vi "DIO tester.vi"() -> ()   [LabVIEW 2013]
uses:
  <vilib>/rvi/Emulation/niFpgaSctlEmulationGetInTimedLoop.vi
  <vilib>/rvi/Emulation/niFpgaEmulationReportErrorSimple.vi
  <vilib>/rvi/Emulation/niFpgaGetClockAttributes.vi
  <vilib>/rvi/eio/common/nirviEmuTemplateMethod_errors.vi
  <vilib>/rvi/Emulation/niFpgaCriticalErrorInLSC.vi
  <vilib>/rvi/Emulation/niFpgaProcessEmulError.vi
  <vilib>/eio/EIONode/EIONode.xnode
panel:
  in  "WE":bool
  in  "IO Module\\DIO Port 0 WE":bool
  out "Row bits":u8 format="%.0b"
  out "Column bits":u8 format="%.0b"
  out "bit9":bool
  out "bit8":bool
  out "Port1":u8 format="%.0b"
  out "Port0":u8 format="%.0b"
  in  "auto":bool
  out "Column":u16
  out "Row":u16
  in  "10thIndex":u8
  in  "ActiveLedIndex":u16
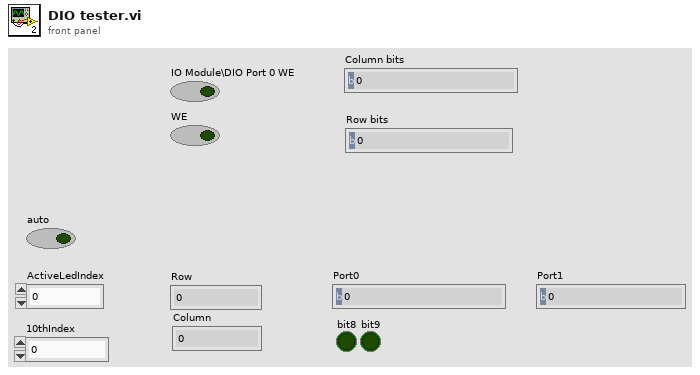
[diagram p1: front panel]
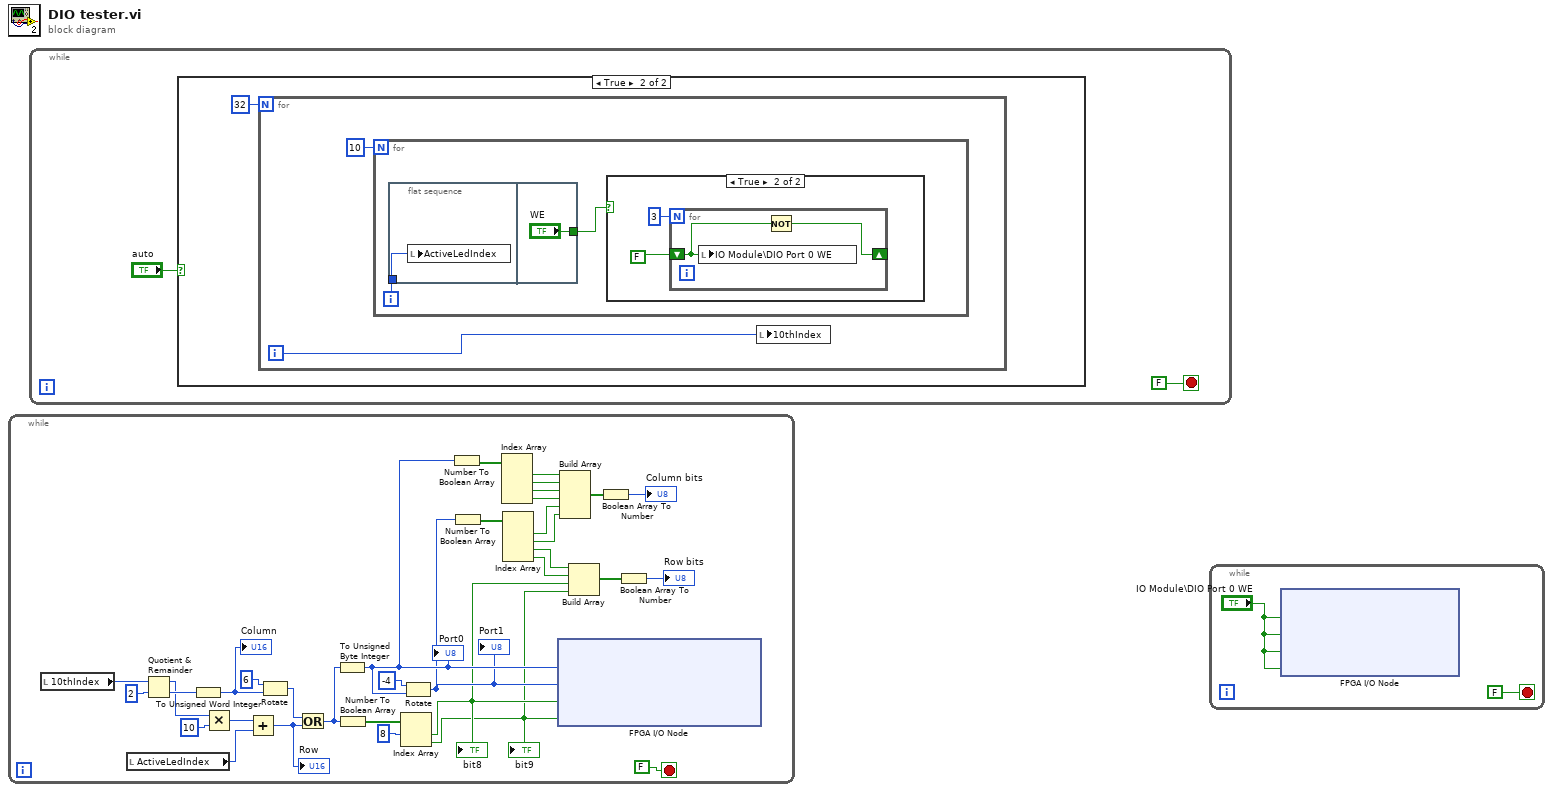
[diagram p0: block diagram]
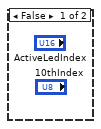
[diagram p2: hidden frame]
diagram:
  n1 = while {
    stop <- FALSE stop-if-true
    n2 = local read "10thIndex"() -> (w24:u8)
    n3 = local read "ActiveLedIndex"() -> (w34:u16)
    n4 = Quotient & Remainder(x=w24, y=u8 2) -> (x-y*floor(x/y)=w21:u8, floor(x/y)=w22:u8)
    n5 = To Unsigned Word Integer(number=w22) -> (unsigned 16bit integer=w28:u16)
    "Column" <- w28
    n6 = Multiply(x=w21, y=u8 10) -> (x*y=w20:u8)
    n7 = Add(x=w20, y=w34) -> (x+y=w32:u16)
    "Row" <- w32
    n8 = Rotate(1:w28, 2:u16 6 ("x")) -> (0:w33:u16)
    n9 = Or(x=w33, y=w32) -> (x .or. y?=w31:u16)
    n10 = To Unsigned Byte Integer(number=w31) -> (unsigned 8bit integer=w18:u8)
    "Port0" <- w18
    n11 = Number To Boolean Array(number=w31) -> (Boolean array=w30:bool[])
    n12 = Index Array(array=w30, index #1=8 ("index")) -> (element #1=w4:bool, element #2=w3:bool)  [unwired: 1 in]
    "bit8" <- w4
    "bit9" <- w3
    n13 = Rotate(1:w18, 2:i16 -4 ("y")) -> (0:w17:u8)
    "Port1" <- w17
    n14 = Number To Boolean Array(number=w18) -> (Boolean array=w16:bool[])
    n15 = Number To Boolean Array(number=w17) -> (Boolean array=w15:bool[])
    n16 = Index Array(array=w16) -> (element #1=w14:bool, element #2=w13:bool, element #3=w12:bool, element #4=w11:bool)  [unwired: 4 in]
    n17 = Index Array(array=w15) -> (element #1=w10:bool, element #2=w9:bool, element #3=w6:bool, element #4=w5:bool)  [unwired: 4 in]
    n18 = xnode "FPGA I/O Node"("IO Module\\DIO Port 0 Wr Data"=w18, "IO Module\\DIO Port 1 Wr Data"=w17, "IO Module\\PFI 0 Wr Data"=w4, "IO Module\\PFI 1 Wr Data"=w3) -> ()  [unwired: 4 in, 4 out]
    n19 = Build Array(w14, w13, w12, w11, w10, w9) -> (w8:bool[])
    n20 = Build Array(w6, w5, w4, w3) -> (w2:bool[])
    n21 = Boolean Array To Number(Boolean array=w8) -> (number=→"Column bits":u8)
    n22 = Boolean Array To Number(Boolean array=w2) -> (number=→"Row bits":u8)
  }
  n23 = while {
    stop <- FALSE stop-if-true
    n24 = case shown="True" "auto" {
      frame False {
      }
      frame True {
        n25 = for {
          N: 32 -> [_]
          i -> [w38]
          n26 = for {
            N: 10 -> [_]
            i -> [w41]
            n27 = flat-sequence {
              tunnel: w41 -> [w42]
              tunnel: ["WE"] -> w40
              frame #0 {
                n28 = local write "ActiveLedIndex"(w42) -> ()
              }
              frame #1 {
              }
            }
            n29 = case shown="True" w40 {
              frame False {
              }
              frame True {
                n30 = for {
                  N: 3 -> [_]
                  shift-right: [w46] -> _
                  shift-left: FALSE -> [w47]
                  n31 = local write "IO Module\\DIO Port 0 WE"(w47) -> ()
                  n32 = Not(x=w47) -> (.not. x?=w46:bool)
                }
              }
            }
          }
          n33 = local write "10thIndex"(w38) -> ()
        }
      }
    }
  }
  n34 = while {
    stop <- FALSE stop-if-true
    n35 = xnode "FPGA I/O Node"("IO Module\\DIO Port 0 WE"="IO Module\\DIO Port 0 WE", "IO Module\\DIO Port 1 WE"="IO Module\\DIO Port 0 WE", "IO Module\\PFI 0 WE"="IO Module\\DIO Port 0 WE", "IO Module\\PFI 1 WE"="IO Module\\DIO Port 0 WE") -> ()  [unwired: 4 in, 4 out]
  }
